vi "PC_Pub_imgFile updFileData.vi"(8 "error in (no error)":errorcluster, 10 "dataName":string, 11 "imgFile in":refnum<class "PC_Pub_imgFile.lvclass">) -> (0 "error out":errorcluster, 3 "imgFile out":refnum<class "PC_Pub_imgFile.lvclass">)   [LabVIEW 2018, in "PC_Pub_imgFile.lvclass"]
uses:
  PC_Pub_imgFile.lvclass
  PC_Pub_imgFile.lvclass/PC_Pub_imgFile.ctl
  <vilib>/zip/NI_Unzip.lvlib
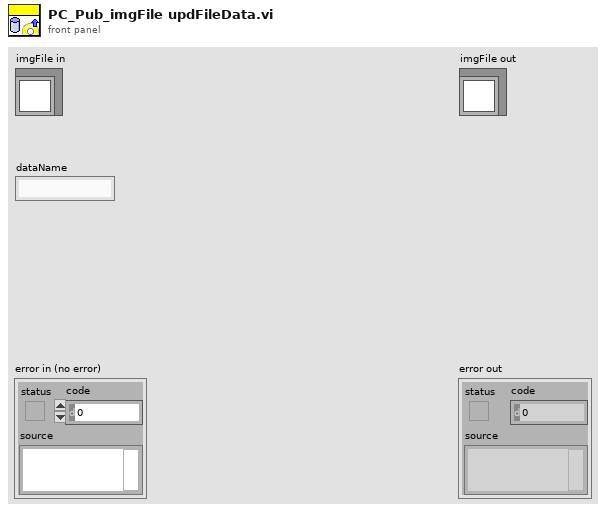
[diagram p1: front panel]
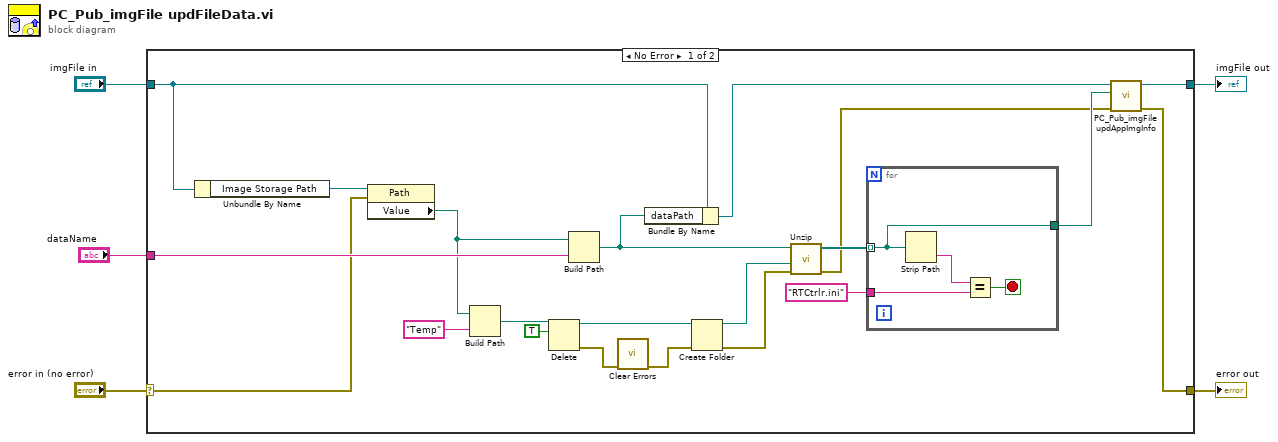
[diagram p0: block diagram]
diagram:
  n1 = case shown="No Error" "error in (no error)" {
    selector: "error in (no error)" -> [w24 w32]
    tunnel: [w9 w32] -> w4
    tunnel: [w12 w31] -> w2
    tunnel: "imgFile in" -> [w8 w31]
    tunnel: "dataName" -> [w25 _]
    frame No Error {
      n2 = Unbundle By Name(w8) -> ("Image Storage Path"=w26:refnum<vi>)
      n3 = property class="Path"(reference=w26, error in=w24) -> ("Value"=w23:path)  [unwired: 2 out]
      n4 = Build Path(base path=w23, name or relative path="Temp") -> (appended path=w21:path)
      n5 = Delete(path (use dialog)=w21, entire hierarchy (F)=TRUE) -> (deleted path=w19:path, error out=w18:errorcluster)  [unwired: 3 in, 1 out]
      n6 = Build Path(base path=w23, name or relative path=w25) -> (appended path=w7:path)
      n7 = call <vilib>:"Clear Errors.vi"("error in (no error)"=w18) -> ("error out"=w17:errorcluster)  [unwired: 5 in, 1 out]
      n8 = Bundle By Name(cluster=w8, "dataPath"=w7) -> (w6:refnum<class "PC_Pub_imgFile.lvclass">)
      n9 = Create Folder(path (use dialog)=w19, error in=w17) -> (created path=w16:path, error out=w11:errorcluster)  [unwired: 1 in, 1 out]
      n10 = call <vilib>:"Unzip.vi"("error in (no error)"=w11, "Target directory (same as Zip file if empty)"=w16, "Zip file"=w7) -> ("error out"=w10:errorcluster, "Unzipped files"=w15:path[])  [unwired: 6 in, 1 out]
      n11 = for {
        tunnel: w15 -> [w27] mode=indexing
        tunnel: "RTCtrlr.ini" -> [w29]
        tunnel: [w27] -> w13
        stop <- w28 stop-if-true
        n12 = Strip Path(path=w27) -> (name=w30:string)  [unwired: 1 out]
        n13 = Equal?(x=w30, y=w29) -> (x = y?=w28:bool)
      }
      n14 = call "PC_Pub_imgFile updAppImgInfo.vi"("error in (no error)"=w10, "RTCtrlrPath"=w13, "imgFile in"=w6) -> ("error out"=w9:errorcluster, "imgFile out"=w12:refnum<class "PC_Pub_imgFile.lvclass">)  [unwired: 7 in]
    }
    frame Error {
    }
  }
  "error out" <- w4
  "imgFile out" <- w2
